vi "writeToXML.vi"(8 "error in (no error)":errorcluster, 10 "classLabel":string, 11 "ShutDown in":refnum<class "ShutDown.lvclass">) -> (0 "error out":errorcluster, 2 "XML out":string, 3 "ShutDown out":refnum<class "ShutDown.lvclass">)   [LabVIEW 2014, in "TCSDataDefinitions.lvlib" / "TCSCommand.lvlib" / "ShutDown.lvclass"]
uses:
  ShutDown.lvclass
  TCSTcsCommand/TCSTcsCommand.lvclass
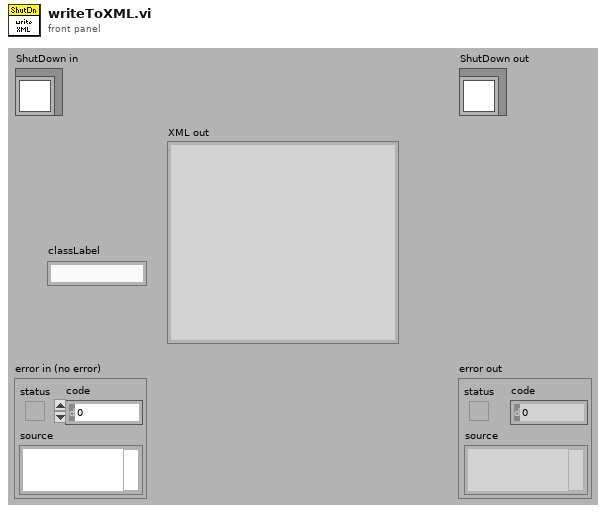
[diagram p1: front panel]
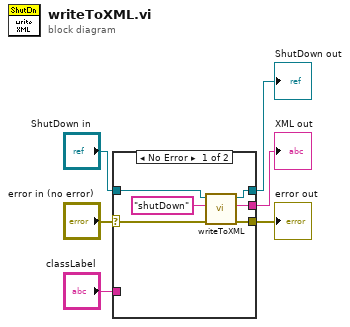
[diagram p0: block diagram]
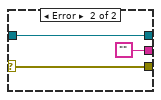
[diagram p2: hidden frame]
diagram:
  n1 = case shown="No Error" "error in (no error)" {
    selector: "error in (no error)" -> [w11 w15]
    tunnel: [w10 w15] -> w5
    tunnel: [w7 w14] -> w3
    tunnel: "ShutDown in" -> [w8 w14]
    tunnel: [w9 ""] -> w2
    tunnel: "classLabel" -> [_ _]
    frame No Error {
      n2 = call-parent "writeToXML.vi"("error in (no error)"=w11, "ClassLabel"="shutDown", "TCSTcsCommand in"=w8) -> ("error out"=w10:errorcluster, "XML out"=w9:string, "TCSTcsCommand out"=w7:refnum<class "ShutDown.lvclass">)  [unwired: 6 in]
    }
    frame Error {
    }
  }
  "error out" <- w5
  "ShutDown out" <- w3
  "XML out" <- w2
